vi "Gain&Offset to Hi&Lo Voltages.vi"(9 "AmpGain":i32=1, 10 "AWG Offset":dbl, 11 "AWG Gain":dbl=1.0) -> (2 "VLo":dbl, 3 "VHi":dbl)   [LabVIEW 2013]
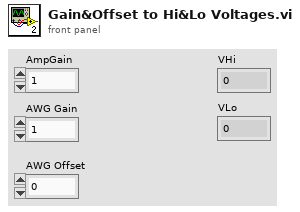
[diagram p1: front panel]
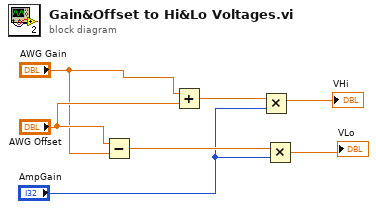
[diagram p0: block diagram]
diagram:
  n1 = Subtract(x="AWG Offset", y="AWG Gain") -> (x-y=w4:dbl)
  n2 = Add(x="AWG Gain", y="AWG Offset") -> (x+y=w6:dbl)
  n3 = Multiply(x=w6, y="AmpGain") -> (x*y=→"VHi":dbl)
  n4 = Multiply(x=w4, y="AmpGain") -> (x*y=→"VLo":dbl)
